vi "Format Numbers.vi"(10 "Precision in":i16[](array[numeric]), 11 "Number In":dbl[](array[numeric])) -> (3 "String out":string[](array[string]))   [LabVIEW 2017]
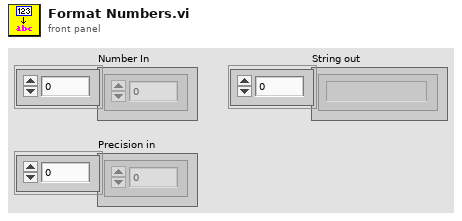
[diagram p1: front panel]
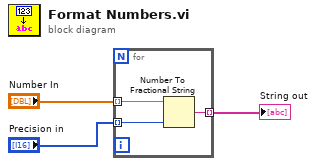
[diagram p0: block diagram]
diagram:
  n1 = for {
    tunnel: [w6] -> w3 mode=indexing
    tunnel: "Number In" -> [w5] mode=indexing
    tunnel: "Precision in" -> [w4] mode=indexing
    n2 = Number To Fractional String(number=w5, precision (6)=w4) -> (F-format string=w6:string)  [unwired: 2 in]
  }
  "String out" <- w3
